vi "PI_Controller.vi"() -> ()   [LabVIEW 2013]
panel:
  in  "Coldfinger\nTemperature (K)":dbl=77.0
  in  "Proportional":dbl=3.0
  in  "Integral":dbl
  in  "Heater Current":u16(ring) items=["Low", "Medium", "High"]
  out "Waveform Chart":dbl(graph)
  out "Percentage \nHeater \nOutput":dbl(knob) scale=0.0..100.0
  in  "?":bool
  out "Temperature (K)":dbl
  in  "dt (s)":dbl=0.5
  in  "Temperature \nSetpoint (K)":dbl=100.0
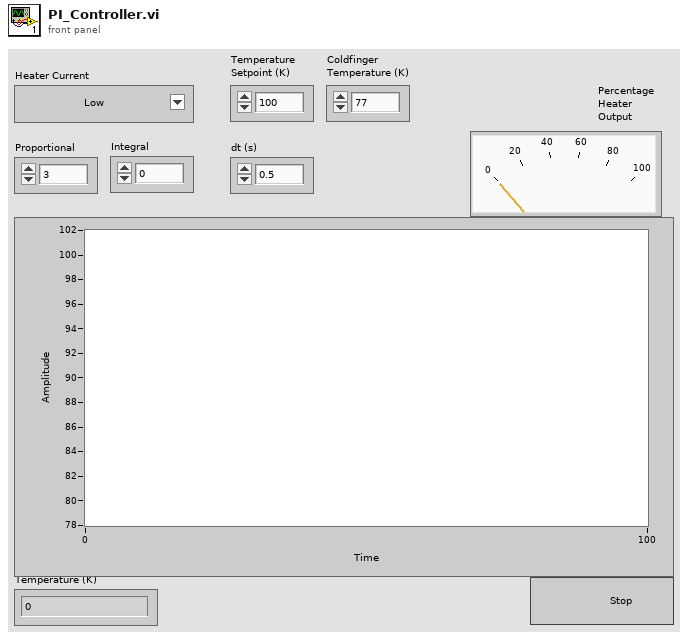
[diagram p1: front panel]
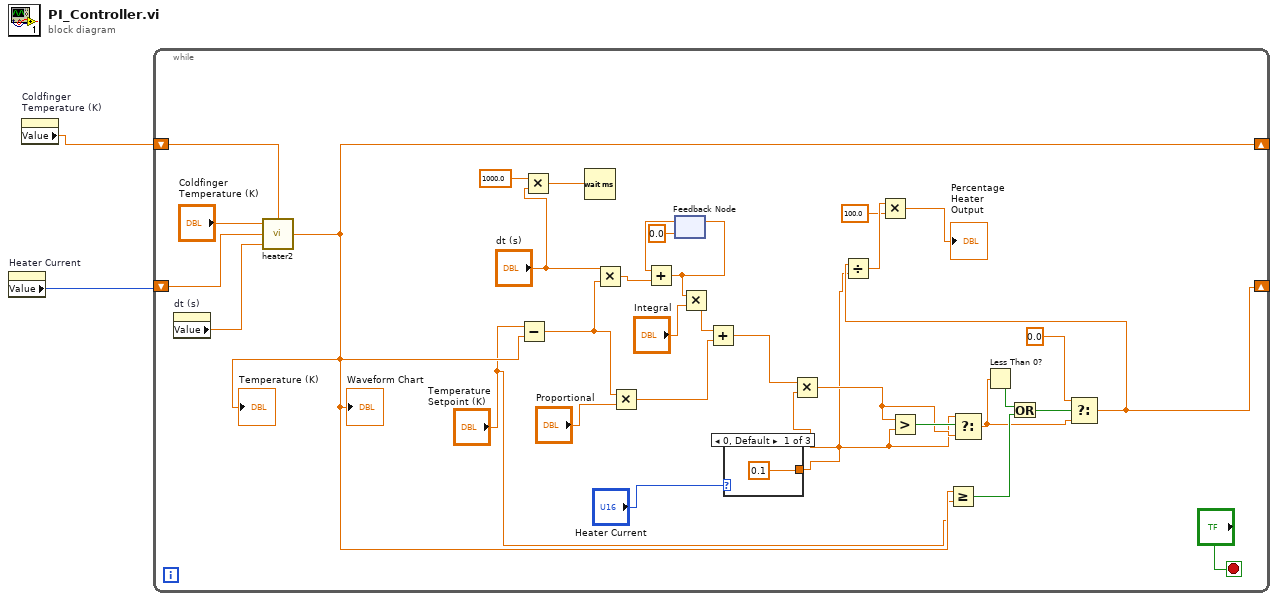
[diagram p0: block diagram]
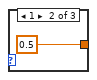
[diagram p2: hidden frame]
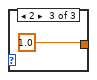
[diagram p3: hidden frame]
diagram:
  n1 = property on="Heater Current" class="Ring (strict)"() -> ("Value"=w2:u16)  [unwired: 2 in, 2 out]
  n2 = property on="Coldfinger\nTemperature (K)" class="DigNum (strict)"() -> ("Value"=w1:dbl)  [unwired: 2 in, 2 out]
  n3 = while {
    shift-right: [w7] -> _
    shift-left: w2 -> [w23]
    shift-right: [w15] -> _
    shift-left: w1 -> [w21]
    stop <- "?" stop-if-true
    n4 = property on="dt (s)" class="DigNum (strict)"() -> ("Value"=w22:dbl)  [unwired: 2 in, 2 out]
    n5 = call "heater2.vi"("Tin"=w21, "dt (seconds)"=w22, "Current"=w23, "Tamb"="Coldfinger\nTemperature (K)") -> ("Tout"=w15:dbl)
    "Temperature (K)" <- w15
    "Waveform Chart" <- w15
    n6 = Subtract(x="Temperature \nSetpoint (K)", y=w15) -> (x-y=w32:dbl)
    n7 = Multiply(x=sgl 1000.0, y="dt (s)") -> (x*y=w8:dbl)
    n8 = Wait (ms)(milliseconds to wait=w8) -> ()  [unwired: 1 out]
    n9 = Multiply(x="dt (s)", y=w32) -> (x*y=w31:dbl)
    n10 = Multiply(x=w32, y="Proportional") -> (x*y=w26:dbl)
    n11 = feedback #1(0.0) -> (w30:dbl)
    n12 = Add(x=w30, y=w31) -> (x+y=w28:dbl)
    n13 = feedback-in #1(w28) -> ()
    n14 = Multiply(x=w28, y="Integral") -> (x*y=w25:dbl)
    n15 = Add(x=w25, y=w26) -> (x+y=w24:dbl)
    n16 = case shown="0, Default" "Heater Current" {
      tunnel: [0.1 0.5 1.0] -> w6
      frame 0, Default {
      }
      frame 1 {
      }
      frame 2 {
      }
    }
    n17 = Multiply(x=w24, y=w6) -> (x*y=w18:dbl)
    n18 = Greater?(x=w18, y=w6) -> (0:w19:bool)
    n19 = Greater Or Equal?(x=w15, y="Temperature \nSetpoint (K)") -> (x >= y?=w16:bool)
    n20 = Select(t=w6, s=w19, f=w18) -> (s? t:f=w11:dbl)
    n21 = Less Than 0?(x=w11) -> (x < 0?=w17:bool)
    n22 = Or(x=w17, y=w16) -> (x .or. y?=w13:bool)
    n23 = Select(t=0.0, s=w13, f=w11) -> (s? t:f=w7:dbl)
    n24 = Divide(x=w7, y=w6) -> (x/y=w5:dbl)
    n25 = Multiply(x=w5, y=100.0) -> (x*y=→"Percentage \nHeater \nOutput":dbl)
  }
